vi "Log Stim Data.vi"(3 "Data Channel":T1) -> ()   [LabVIEW 2019]
uses:
  <extravilib>/ChannelInstances/Messenger-t'Log Message.ctl'/))Channel.ctl
  Lee Lab/CP FES Walking 2018/Code/Working/LabVIEW/Controls/Messages/Log Message.ctl
  Lee Lab/CP FES Walking 2018/Code/Working/LabVIEW/Controls/States/Log State.ctl
  <extravilib>/ChannelInstances/Messenger-t'Log Message.ctl'/Read With Abort.vi
  <resource>/Channels/Messenger/Read With Abort.vi
  <vilib>/ChannelSupport/Channel Message/Read ID.vi
  <resource>/Channels/Messenger/Endpoint.vi
  <extravilib>/ChannelInstances/Messenger-t'Log Message.ctl'/Unwrap.vi
  <extravilib>/ChannelInstances/Messenger-t'Log Message.ctl'.lvlib
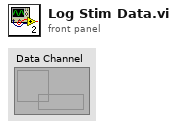
[diagram p1: front panel]
types:
  T1 = typedef "Messenger-t'Log Message.ctl'.lvlib/))Channel.ctl" = refnum<queue>
  T2 = typedef "Log Message.ctl" = cluster{"Log State":T3, "Data":variant}
  T3 = typedef "Log State.ctl" = enum16{"Open", "Initialize", "Update", "On", "Off", "Idle", "Close", "Quit"}
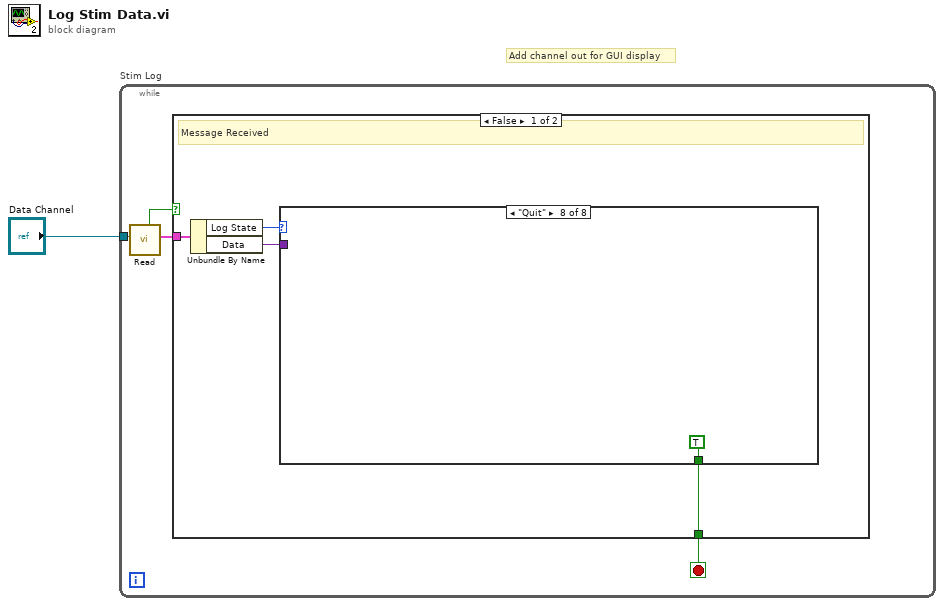
[diagram p0: block diagram]
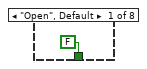
[diagram p2: hidden frame]
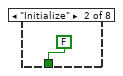
[diagram p3: hidden frame]
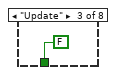
[diagram p4: hidden frame]
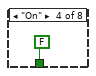
[diagram p5: hidden frame]
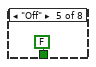
[diagram p6: hidden frame]
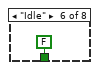
[diagram p7: hidden frame]
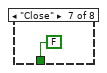
[diagram p8: hidden frame]
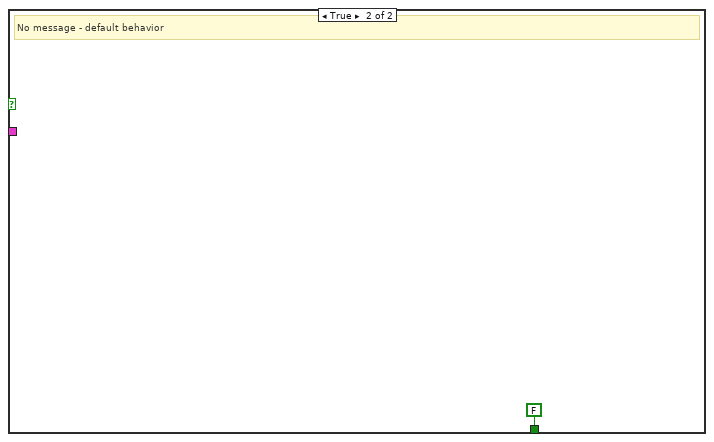
[diagram p9: hidden frame]
diagram:
  # "Add channel out for GUI display"
  n1 = while "Stim Log" {
    tunnel: "Data Channel" -> [w4]
    stop <- w5 stop-if-true
    n2 = call <extravilib>:"Read.vi"("channel"=w4) -> ("element"=w3:T2, "timedout?"=w2:bool)  [unwired: 7 in, 2 out]
    n3 = case shown="False" w2 {
      tunnel: [w9 FALSE] -> w5
      tunnel: w3 -> [w6 _]
      frame False {
        # "Message Received"
        n4 = Unbundle By Name(w6) -> ("Log State"=w8:T3, "Data"=w7:variant)
        n5 = case shown="\"Quit\"" w8 {
          tunnel: w7 -> [_ _ _ _ _ _ _ _]
          tunnel: [FALSE FALSE FALSE FALSE FALSE FALSE FALSE TRUE] -> w9
          frame "Open", Default {
          }
          frame "Initialize" {
          }
          frame "Update" {
          }
          frame "On" {
          }
          frame "Off" {
          }
          frame "Idle" {
          }
          frame "Close" {
          }
          frame "Quit" {
          }
        }
      }
      frame True {
        # "No message - default behavior"
      }
    }
  }
